vi "stdVisitorTimeout.vi"(3 "Agent ID":string, 4 "standard Visitor":T1) -> (0 "stdVisit?":bool, 1 "dup HGF_NetworkData":refnum<class "HGF_NetworkVisitor.lvclass">, 2 "error out":errorcluster)   [LabVIEW 2009, in "MoAgSy.lvlib" / "MoAgSy_Engine.lvclass"]
uses:
  MoAgSy_Engine.lvclass
  Visitors/MoAgSy_Visitor/MoAgSy_Visitor.lvclass
  HGF_BaseClasses/HGF_NetworkVisitor/HGF_NetworkVisitor.lvclass
  MoAgSy_Factory/MoAgSy_Factory.lvclass
  HGF_BaseClasses/HGF_Factory/HGF_Factory.lvclass
  MoAgSy_Message/MoAgSy_Message.lvclass
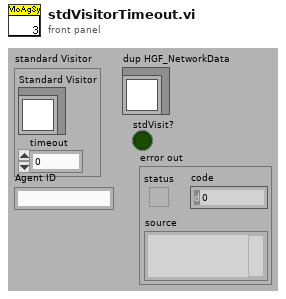
[diagram p1: front panel]
types:
  T1 = cluster{"Standard Visitor":refnum<class "MoAgSy_Visitor.lvclass">, "timeout":dbl}
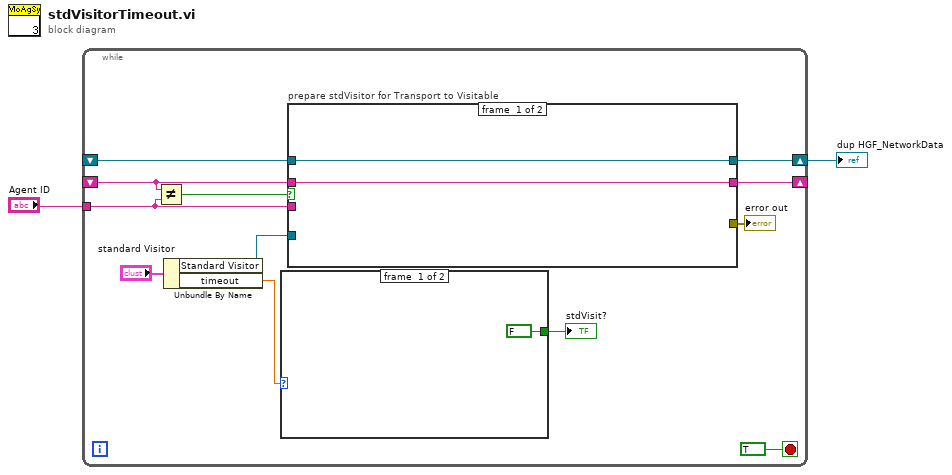
[diagram p0: block diagram]
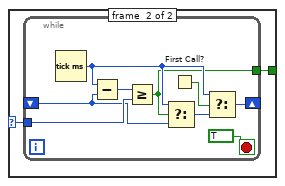
[diagram p2: hidden frame]
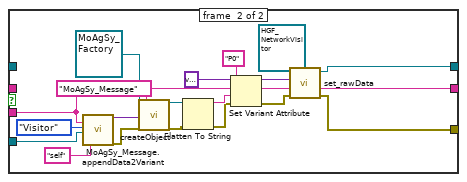
[diagram p3: hidden frame]
diagram:
  n1 = while {
    shift-right: [w10] -> w2
    shift-left: _ -> [w9]
    tunnel: "Agent ID" -> [w7]
    shift-right: [w8] -> _
    shift-left: _ -> [w5]
    stop <- TRUE stop-if-true
    n2 = Not Equal?(x=w5, y=w7) -> (x != y?=w6:bool)
    n3 = Unbundle By Name("standard Visitor") -> ("Standard Visitor"=w13:refnum<class "MoAgSy_Visitor.lvclass">, "timeout"=w11:dbl)
    n4 = case shown="0, Default" w11 {
      selector: w11 -> [_ w16]
      tunnel: [FALSE w17] -> w12
      frame #0 {
      }
      frame #1 {
        n5 = while {
          tunnel: w16 -> [w24]
          shift-right: [w20] -> _
          shift-left: _ -> [w23]
          tunnel: [w18] -> w17
          stop <- TRUE stop-if-true
          n6 = Tick Count (ms)() -> (millisecond timer value=w22:u32)
          n7 = Subtract(x=w22, y=w23) -> (x-y=w25:u32)
          n8 = Greater Or Equal?(x=w25, y=w24) -> (x >= y?=w18:bool)
          n9 = Select(t=w22, s=w18, f=w23) -> (s? t:f=w19:u32)
          n10 = First Call?() -> (First Call?: T/F=w21:bool)
          n11 = Select(t=w22, s=w21, f=w19) -> (s? t:f=w20:u32)
        }
      }
    }
    "stdVisit?" <- w12
    n12 = case "prepare stdVisitor for Transport to Visitable" shown="True" w6 {
      tunnel: w13 -> [_ w44]
      tunnel: [w28 w34] -> w10
      tunnel: w9 -> [w28 _]
      tunnel: w7 -> [_ w33]
      tunnel: [w27 w33] -> w8
      tunnel: w5 -> [w27 _]
      tunnel: [_ w29] -> w3
      frame #0 {
      }
      frame #1 {
        n13 = call "MoAgSy_Message.appendData2Variant.vi"("addressee"=w33, "type"=enum16{"mobile Agent", "Visitor", "Message"}."Visitor", "Object"=w44, "sender"="self") -> ("dup_initData"=w47:variant, "error out"=w30:errorcluster)  [unwired: 14 in]
        n14 = call "createObject.vi"("HGF_Factory"=refnum<class "MoAgSy_Factory.lvclass"> refnum ("MoAgSy.lvlib:MoAgSy_Factory.lvclass"), "initializationData"=w47, "error in (no error)"=w30, "className"="MoAgSy_Message") -> ("HGF_Object"=w39:refnum<class "HGF_Factory.lvclass">, "error out"=w40:errorcluster)  [unwired: 13 in, 1 out]
        n15 = Flatten To String(anything=w39, error in (no error)=w40) -> (data string=w36:string, error out=w32:errorcluster)  [unwired: 2 in, 1 out]
        n16 = Set Variant Attribute(Variant=variant ("rawData"), name="P0", value=w36, error in=w32) -> (Variant out=w37:variant, error out=w31:errorcluster)  [unwired: 1 out]
        n17 = call "set_rawData.vi"("error in (no error)"=w31, "rawData"=w37, "HGF_NetworkData"=refnum<class "HGF_NetworkVisitor.lvclass"> refnum ("HGF_BaseClasses.lvlib:HGF_NetworkVisitor.lvclass")) -> ("error out"=w29:errorcluster, "dup HGF_NetworkData"=w34:refnum<class "HGF_NetworkVisitor.lvclass">)  [unwired: 7 in]
      }
    }
    "error out" <- w3
  }
  "dup HGF_NetworkData" <- w2
